vi "Get_fast_sequences.vi"(1 "Doubles":dbl[](array[numeric]), 2 "Array":dbl[][](array[numeric])) -> (0 "Fast sequence":T7(array[cluster]) {"DAC"."DAC offset" min=-1 max=0.5; "DAC"."FastChanNum" max=15 step=1; "slot#" max=4095})   [LabVIEW 2013]
uses:
  sequence slot/slot-use.ctl
  sequence slot/triggers.ctl
  sequence slot/DAC.ctl
  sequence slot/DAC_fastseq-offset.ctl
  sequence slot/timing.ctl
  sequence slot/jump.ctl
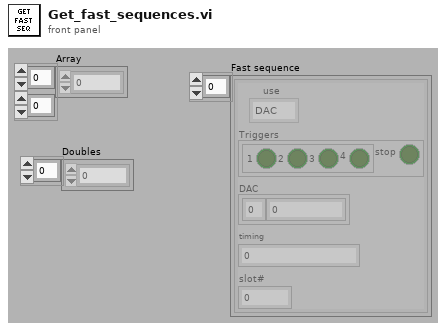
[diagram p1: front panel]
types:
  T1 = typedef "slot-use.ctl" = enum8{"DAC", "timing", "triggers", "jump"}
  T2 = typedef "triggers.ctl" = cluster{"triggers":cluster{"1":bool, "2":bool, "3":bool, "4":bool}, "stop":bool}
  T3 = typedef "DAC.ctl" = cluster{"FastChanNum":u8, "DAC offset":T4}
  T4 = typedef "DAC_fastseq-offset.ctl" = sgl
  T5 = typedef "timing.ctl" = sgl
  T6 = typedef "jump.ctl" = u16
  T7 = cluster{"use":T1, "Triggers":T2, "DAC":T3, "timing":T5, "slot#":T6}[]
  T8 = cluster{"use":T1, "Triggers":T2, "DAC":T3, "timing":T5, "slot#":T6}
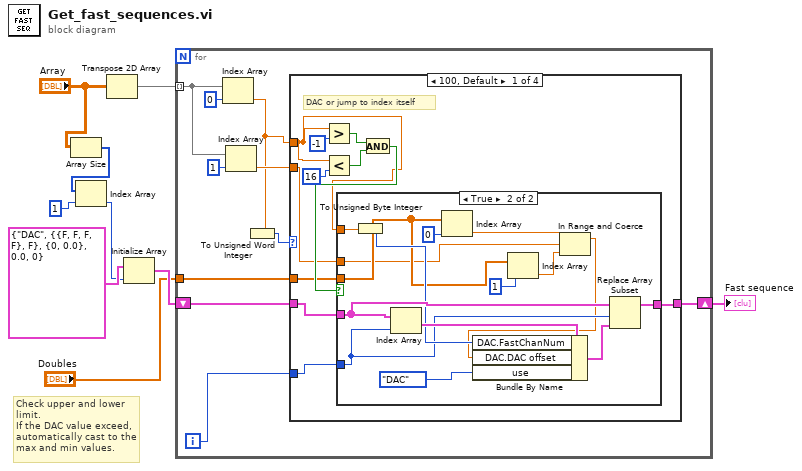
[diagram p0: block diagram]
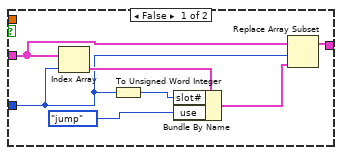
[diagram p2: hidden frame]
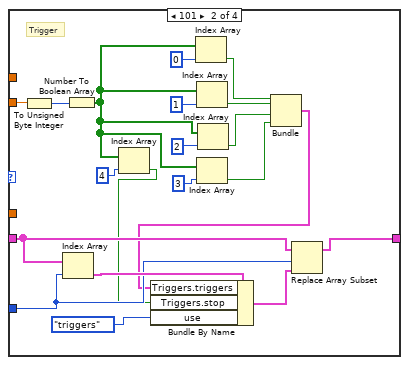
[diagram p3: hidden frame]
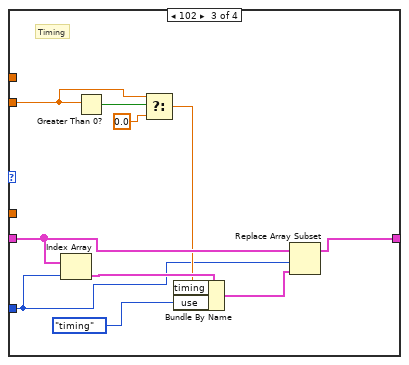
[diagram p4: hidden frame]
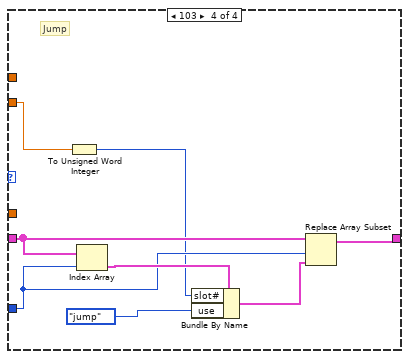
[diagram p5: hidden frame]
diagram:
  # "Check upper and lower\nlimit.\nIf the DAC value exceed,\nautomatically cast to the\nmax and min values."
  n1 = Array Size(array="Array") -> (size(s)=w7:i32[])
  n2 = Index Array(array=w7, index=1) -> (element=w4:i32)
  n3 = Transpose 2D Array(2D array="Array") -> (transposed array=w9:dbl[][])
  n4 = Initialize Array(T8 {"use"=enum."DAC", "Triggers"={"triggers"={"1"=FALSE, "2"=FALSE, "3"=FALSE, "4"=FALSE}, "stop"=FALSE}, "DAC"={"FastChanNum"=0, "DAC offset"=0.0}, "timing"=0.0, "slot#"=0} ("slot 0"), w4) -> (w3:T7)
  n5 = for {
    tunnel: w9 -> [w14] mode=indexing
    shift-right: [w12] -> w1
    shift-left: w3 -> [w17]
    tunnel: "Doubles" -> [w11]
    i -> [w16]
    n6 = Index Array(array=w14, index=0) -> (element=w10:dbl)
    n7 = Index Array(array=w14, index=1) -> (element=w13:dbl)
    n8 = To Unsigned Word Integer(number=w10) -> (unsigned 16bit integer=w18:u16)
    n9 = case shown="100, Default" w18 {
      tunnel: w10 -> [w20 _ _ _]
      tunnel: w17 -> [w25 w67 w80 w87]
      tunnel: w16 -> [w24 w65 w73 w85]
      tunnel: w13 -> [w22 w72 w77 w84]
      tunnel: [w23 w66 w74 w86] -> w12
      tunnel: w11 -> [w21 _ _ _]
      frame 100, Default {
        # "DAC or jump to index itself"
        n10 = Greater?(x=w20, y=-1) -> (0:w30:bool)
        n11 = Less?(x=w20, y=16) -> (x < y?=w29:bool)
        n12 = And(x=w30, y=w29) -> (x .and. y?=w26:bool)
        n13 = case shown="True" w26 {
          tunnel: w25 -> [w35 w48]
          tunnel: w24 -> [w32 w43]
          tunnel: w20 -> [_ w52]
          tunnel: [w31 w44] -> w23
          tunnel: w22 -> [_ w39]
          tunnel: w21 -> [_ w46]
          frame False {
            n14 = Index Array(array=w35, index=w32) -> (element=w34:T8)
            n15 = To Unsigned Word Integer(number=w32) -> (unsigned 16bit integer=w33:u16)
            n16 = Bundle By Name(cluster=w34, "slot#"=w33, "use"=slot-use."jump") -> (w36:T8)
            n17 = Replace Array Subset(array=w35, new element=w36, index=w32) -> (w31:T7)
          }
          frame True {
            n18 = To Unsigned Byte Integer(number=w52) -> (unsigned 8bit integer=w47:u8)
            n19 = Index Array(array=w48, index=w43) -> (element=w49:T8)
            n20 = Index Array(array=w46, index=0) -> (element=w40:dbl)
            n21 = Index Array(array=w46, index=1) -> (element=w41:dbl)
            n22 = In Range and Coerce(upper limit=w40, x=w39, lower limit=w41) -> (coerced(x)=w38:dbl)  [unwired: 1 out]
            n23 = Bundle By Name(cluster=w49, "DAC.FastChanNum"=w47, "DAC.DAC offset"=w38, "use"=slot-use."DAC") -> (w50:T8)
            n24 = Replace Array Subset(array=w48, new element=w50, index=w43) -> (w44:T7)
          }
        }
      }
      frame 101 {
        # "Trigger"
        n25 = To Unsigned Byte Integer(number=w72) -> (unsigned 8bit integer=w71:u8)
        n26 = Index Array(array=w67, index=w65) -> (element=w70:T8)
        n27 = Number To Boolean Array(number=w71) -> (Boolean array=w58:bool[])
        n28 = Index Array(array=w58, index=4) -> (element=w63:bool)
        n29 = Index Array(array=w58, index=0) -> (element=w57:bool)
        n30 = Index Array(array=w58, index=1) -> (element=w56:bool)
        n31 = Index Array(array=w58, index=3) -> (element=w54:bool)
        n32 = Index Array(array=w58, index=2) -> (element=w55:bool)
        n33 = Bundle(w57, w56, w55, w54) -> (w53:cluster{bool, bool, bool, bool})  [unwired: 1 in]
        n34 = Bundle By Name(cluster=w70, "Triggers.triggers"=w53, "Triggers.stop"=w63, "use"=slot-use."triggers") -> (w68:T8)
        n35 = Replace Array Subset(array=w67, new element=w68, index=w65) -> (w66:T7)
      }
      frame 102 {
        # "Timing"
        n36 = Index Array(array=w80, index=w73) -> (element=w79:T8)
        n37 = Greater Than 0?(x=w77) -> (x > 0?=w78:bool)
        n38 = Select(t=w77, s=w78, f=0.0) -> (s? t:f=w75:dbl)
        n39 = Bundle By Name(cluster=w79, "timing"=w75, "use"=slot-use."timing") -> (w81:T8)
        n40 = Replace Array Subset(array=w80, new element=w81, index=w73) -> (w74:T7)
      }
      frame 103 {
        # "Jump"
        n41 = To Unsigned Word Integer(number=w84) -> (unsigned 16bit integer=w83:u16)
        n42 = Index Array(array=w87, index=w85) -> (element=w88:T8)
        n43 = Bundle By Name(cluster=w88, "slot#"=w83, "use"=slot-use."jump") -> (w89:T8)
        n44 = Replace Array Subset(array=w87, new element=w89, index=w85) -> (w86:T7)
      }
    }
  }
  "Fast sequence" <- w1
